vi "New Polymorphic VI.vi"(8 "error in (no error)":errorcluster, 10 "App Refnum":refnum<vi>, 11 "SubVI Refnum":refnum<vi>) -> (0 "error out":errorcluster, 3 "Polymorphic VI Type out":refnum<class "Polymorphic VI Type.lvclass">)   [LabVIEW 2020, in "Peek Window.lvlib" / "Polymorphic VI Type.lvclass"]
uses:
  Polymorphic VI Type.lvclass
  D:/Code/VI-Peek/source/Peek Window/VI Types/Standard VI Type/Standard VI Type.lvclass
  Implementation VI Type/Implementation VI Type.lvclass
  Standard VI Type/Standard VI Type.lvclass
  Standard VI Type/Standard VI Type.lvclass/Standard VI Type.ctl
  Polymorphic VI Type.lvclass/Polymorphic VI Type.ctl
  Standard VI Type/Write App Refnum.vi
  Standard VI Type/Write VI Refnum.vi
  Standard VI Type/Write Full Qualified Name.vi
  Standard VI Type/Write Openable.vi
  Standard VI Type/Write Selectable.vi
  Selected Item Enum.ctl
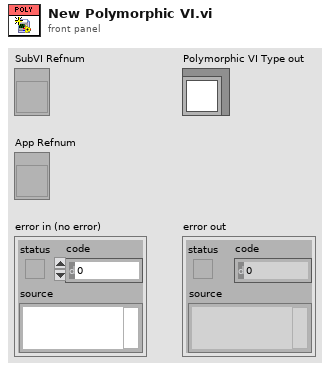
[diagram p1: front panel]
types:
  T1 = typedef "Peek Window.lvlib/Polymorphic VI Type.lvclass/Selected Item Enum.ctl" = enum16{"Polymorphic", "Instance"}
  T2 = map{string, refnum<class "Implementation VI Type.lvclass">}
  T3 = cluster{"VIPath":path, "Menu Name":string, "Selector Name":string}[]
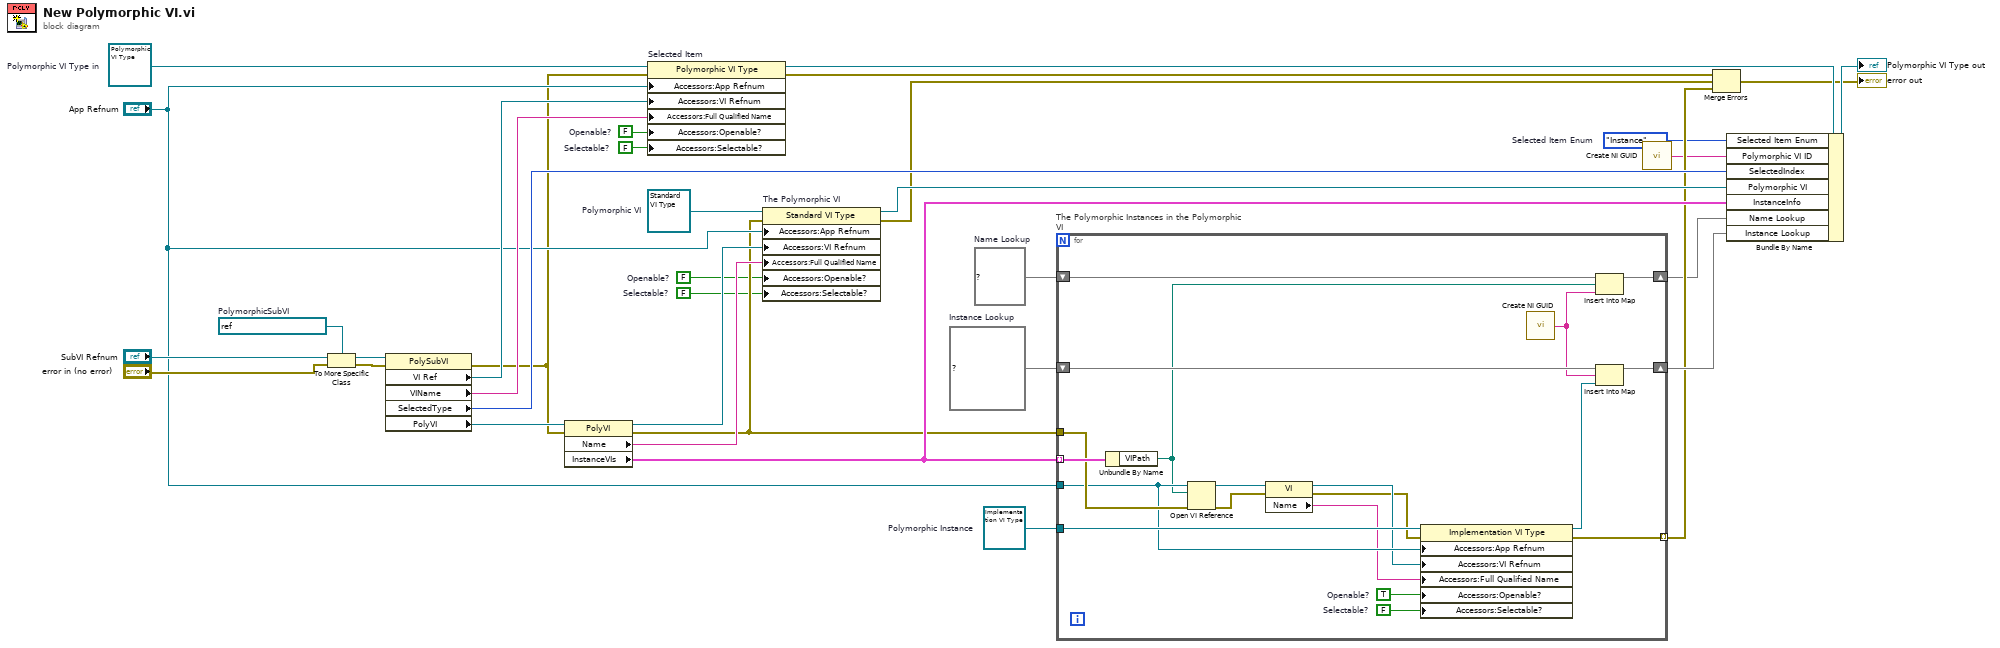
[diagram p0: block diagram]
diagram:
  w1 = Selected_Item_Enum."Instance"  # Selected Item Enum
  w4 = map{path, string} {}  # Name Lookup
  w5 = FALSE  # Selectable?
  w6 = FALSE  # Selectable?
  w7 = FALSE  # Openable?
  w18 = refnum<class "Standard VI Type.lvclass"> refnum  # Polymorphic VI
  w21 = T2 {}  # Instance Lookup
  w19 = refnum<class "Implementation VI Type.lvclass"> refnum  # Polymorphic Instance
  w23 = FALSE  # Openable?
  w32 = refnum<vi> refnum  # PolymorphicSubVI
  w35 = refnum<class "Polymorphic VI Type.lvclass"> refnum  # Polymorphic VI Type in
  n1 = To More Specific Class(target class=w32, reference="SubVI Refnum", error in="error in (no error)") -> (specific class reference=w30:refnum<vi>, error out=w29:errorcluster)
  n2 = property class="PolySubVI"(reference=w30, error in=w29) -> (error out=w11:errorcluster, "VI Ref"=w26:refnum<vi>, "VIName"=w25:string, "SelectedType"=w22:i32, "PolyVI"=w27:refnum<vi>)  [unwired: 1 out]
  n3 = property class="PolyVI"(reference=w27, error in=w11) -> (reference out=w16:refnum<vi>, error out=w13:errorcluster, "Name"=w15:string, "InstanceVIs"=w24:T3)
  n4 = property on="Selected Item" class="Polymorphic VI Type"(reference=w35, error in=w11, "Accessors:App Refnum"="App Refnum", "Accessors:VI Refnum"=w26, "Accessors:Full Qualified Name"=w25, "Accessors:Openable?"=w23, "Accessors:Selectable?"=w6) -> (reference out=w33:refnum<class "Polymorphic VI Type.lvclass">, error out=w10:errorcluster)
  n5 = property on="The Polymorphic VI" class="Standard VI Type"(reference=w18, error in=w13, "Accessors:App Refnum"="App Refnum", "Accessors:VI Refnum"=w16, "Accessors:Full Qualified Name"=w15, "Accessors:Openable?"=w7, "Accessors:Selectable?"=w5) -> (reference out=w17:refnum<class "Standard VI Type.lvclass">, error out=w9:errorcluster)
  n6 = for "The Polymorphic Instances in the Polymorphic VI" {
    tunnel: w24 -> [w54] mode=indexing
    tunnel: w13 -> [w53]
    tunnel: "App Refnum" -> [w48]
    shift-right: [w50] -> w20
    shift-left: w21 -> [w51]
    tunnel: w19 -> [w49]
    tunnel: [w42] -> w12 mode=indexing
    shift-right: [w39] -> w3
    shift-left: w4 -> [w40]
    w41 = FALSE  # Selectable?
    w44 = TRUE  # Openable?
    n7 = Unbundle By Name(w54) -> ("VIPath"=w38:path)
    n8 = Open VI Reference(application reference (local)=w48, vi path=w38, error in (no error)=w53) -> (vi reference=w52:refnum<vi>, error out=w45:errorcluster)  [unwired: 3 in]
    n9 = property class="VI"(reference=w52, error in=w45) -> (reference out=w47:refnum<vi>, error out=w46:errorcluster, "Name"=w37:string)
    n10 = property class="Implementation VI Type"(reference=w49, error in=w46, "Accessors:App Refnum"=w48, "Accessors:VI Refnum"=w47, "Accessors:Full Qualified Name"=w37, "Accessors:Openable?"=w44, "Accessors:Selectable?"=w41) -> (reference out=w43:refnum<class "Implementation VI Type.lvclass">, error out=w42:errorcluster)
    n11 = call <vilib>:"Create NI GUID.vi"() -> ("NI GUID"=w36:string)
    n12 = Insert Into Map(map in=w40, key=w38, value=w36) -> (map out=w39:map{path, string})  [unwired: 2 out]
    n13 = Insert Into Map(map in=w51, key=w36, value=w43) -> (map out=w50:T2)  [unwired: 2 out]
  }
  n14 = call <vilib>:"Create NI GUID.vi"() -> ("NI GUID"=w2:string)
  n15 = Merge Errors(w10, w9, w12) -> (→"error out":errorcluster)
  n16 = Bundle By Name(cluster=w33, "Selected Item Enum"=w1, "Polymorphic VI ID"=w2, "SelectedIndex"=w22, "Polymorphic VI"=w17, "InstanceInfo"=w24, "Name Lookup"=w3, "Instance Lookup"=w20) -> (→"Polymorphic VI Type out":refnum<class "Polymorphic VI Type.lvclass">)
